vi "Read Uml.vi"(8 "error in (no error)":errorcluster, 11 "Class in":refnum<class "Class.lvclass">) -> (0 "error out":errorcluster, 2 "Uml":string, 3 "Class out":refnum<class "Class.lvclass">)   [LabVIEW 2021, in "TAF Proj Document Type.lvlib" / "Class.lvclass"]
uses:
  <vilib>/Wovalab/AntiDoc/Document Type/Add-ons/LabVIEW TAF Project/Class/Class.lvclass
  <vilib>/Wovalab/AntiDoc/Document Type/Add-ons/LabVIEW TAF Project/Class/Class.lvclass/Class.ctl
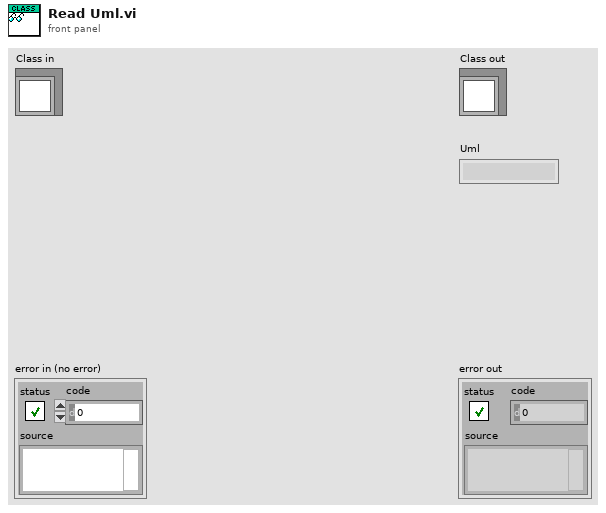
[diagram p1: front panel]
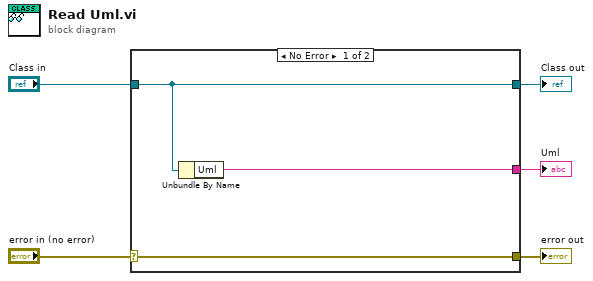
[diagram p0: block diagram]
diagram:
  n1 = case shown="No Error" "error in (no error)" {
    selector: "error in (no error)" -> [w8 w9]
    tunnel: [w8 w9] -> w4
    tunnel: [w7 w10] -> w2
    tunnel: "Class in" -> [w7 w10]
    tunnel: [w6 _] -> w1
    frame No Error {
      n2 = Unbundle By Name(w7) -> ("Uml"=w6:string)
    }
    frame Error {
    }
  }
  "error out" <- w4
  "Class out" <- w2
  "Uml" <- w1
